vi "DMA.Scatter-Gather.Create Block Descriptor.vi"(11 "block":T2 {"size" format="%08x"; "pointer" format="%08x"}) -> (3 "block descriptor":T1 {"next descriptor ptr" format="%08x"; "data size" format="%08x"; "data ptr (upper)" format="%08x"; "data ptr (lower)" format="%08x"; "descriptor ptr (aligned)" format="%08x"; "descriptor size" format="%08x"; "descriptor ptr (VISA)" format="%08x"})   [LabVIEW 2016, in "GE 5565PIORC.lvclass"]
uses:
  GE 5565PIORC.lvclass
  Controls/DMA Block.ctl
  Controls/DMA Block Descriptor.ctl
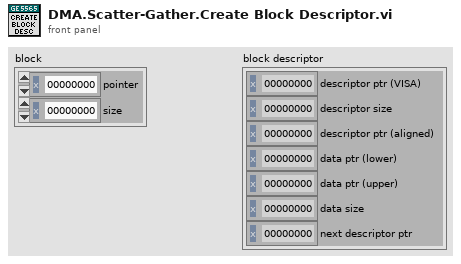
[diagram p1: front panel]
types:
  T1 = typedef "GE 5565PIORC.lvclass/DMA Block Descriptor.ctl" = cluster{"descriptor ptr (VISA)":u32, "descriptor size":u32, "descriptor ptr (aligned)":u32, "data ptr (lower)":u32, "data ptr (upper)":u32, "data size":u32, "next descriptor ptr":u32}
  T2 = typedef "GE 5565PIORC.lvclass/DMA Block.ctl" = cluster{"pointer":u32, "size":u32}
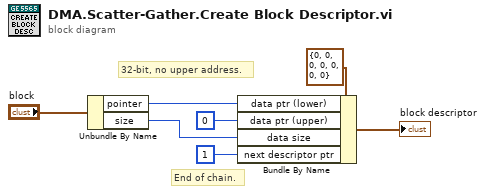
[diagram p0: block diagram]
diagram:
  # "32-bit, no upper address."
  # "End of chain."
  n1 = Unbundle By Name("block") -> ("pointer"=w5:u32, "size"=w1:u32)
  n2 = Bundle By Name(cluster=T1 {"descriptor ptr (VISA)"=0, "descriptor size"=0, "descriptor ptr (aligned)"=0, "data ptr (lower)"=0, "data ptr (upper)"=0, "data size"=0, "next descriptor ptr"=0} ("Block Descriptor"), "data ptr (lower)"=w5, "data ptr (upper)"=u32 0 ("next block pointer"), "data size"=w1, "next descriptor ptr"=u32 1 ("next block pointer")) -> (→"block descriptor":T1)
